vi "ConcidenceTesting.vi"() -> ()   [LabVIEW 2009]
panel:
  in  "new dim":cluster{"x":u32, "y":u32}={"x"=1, "y"=1}
  in  "re-calculate":bool
  in  "Palette Number (gray)":T1(ring)
  in  "coincidence settings":T2={"length [µs]"=10.0, "delayed channel"=0, "center peak (µs)"=0.5, "lateral peaks"=6} {"center peak (µs)" format="%.2f"; "length [µs]" format="%.2f"}
  in  "ratio":bool
  in  "threshold":u32
  in  "calculate":bool
  in  "including +/- Pixel":i32
  in  "stop":bool
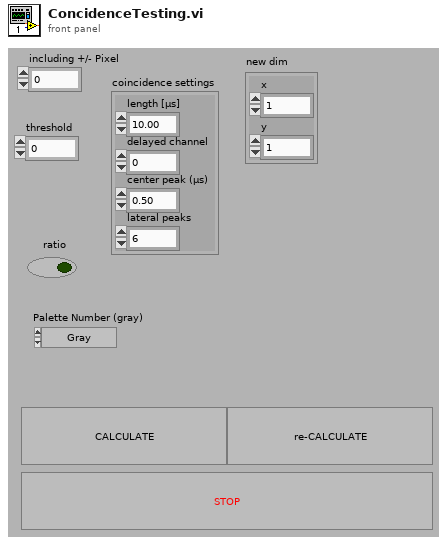
[diagram p1: front panel]
types:
  T1 = enum32{"Gray", "Binary", "Gradient", "Rainbow", "Temperature"}
  T2 = cluster{"length [µs]":dbl, "delayed channel":u8, "center peak (µs)":dbl, "lateral peaks":u32}
  T3 = enum16{"Ini", "Get", "Set", "Draw", "Colorpal", "Dump", "Zoom"}
  T4 = cluster{"router":u8[], "macro times":dbl[], "micro times":u16[], "invalid":dbl[], "gap":dbl[]}
  T5 = cluster{"origin (ns)":dbl, "offset (ns)":dbl, "histogram":u32[]}
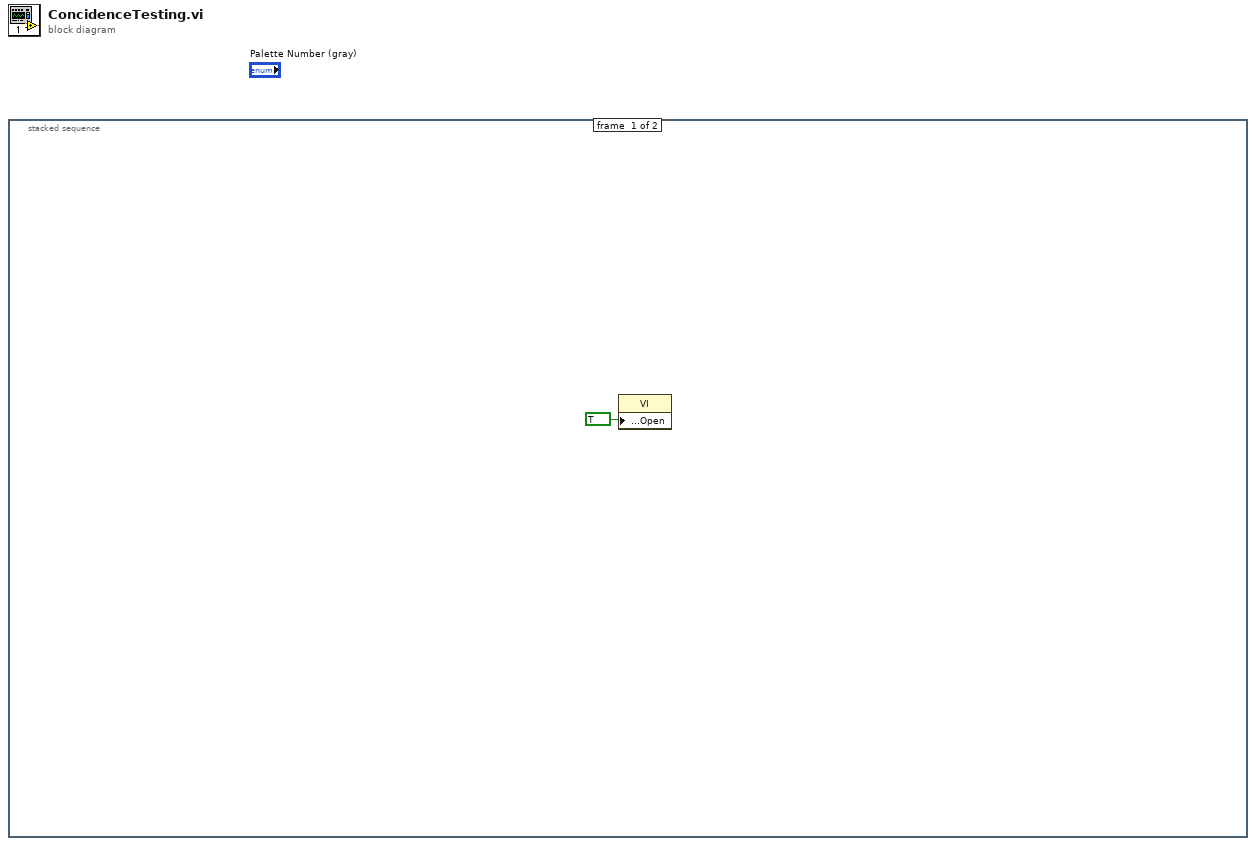
[diagram p0: block diagram]
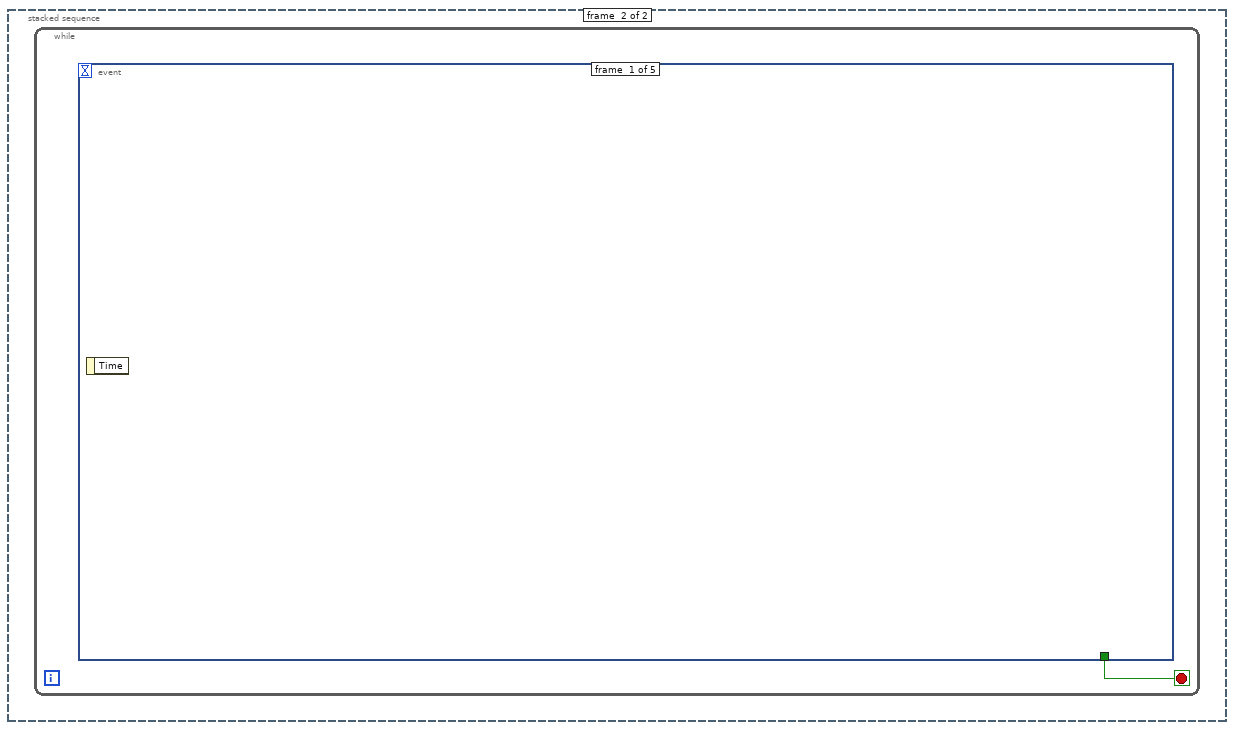
[diagram p2: hidden frame]
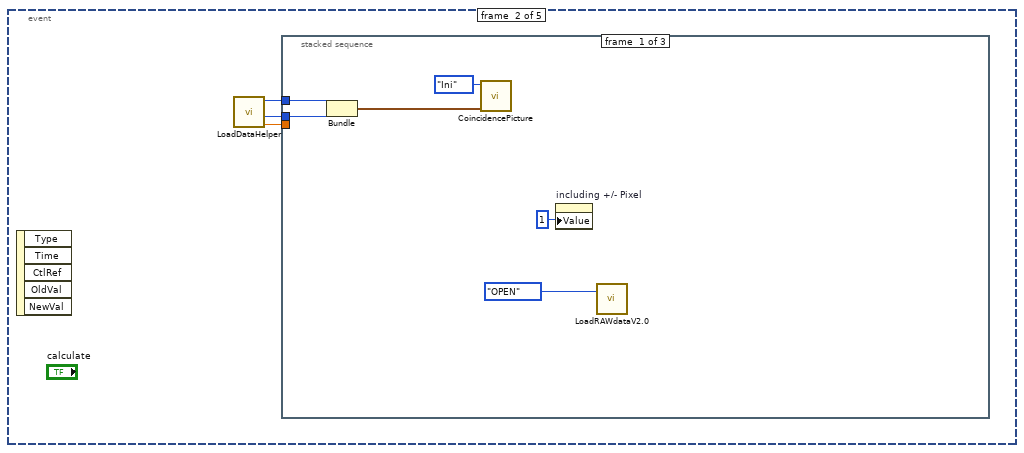
[diagram p3: hidden frame]
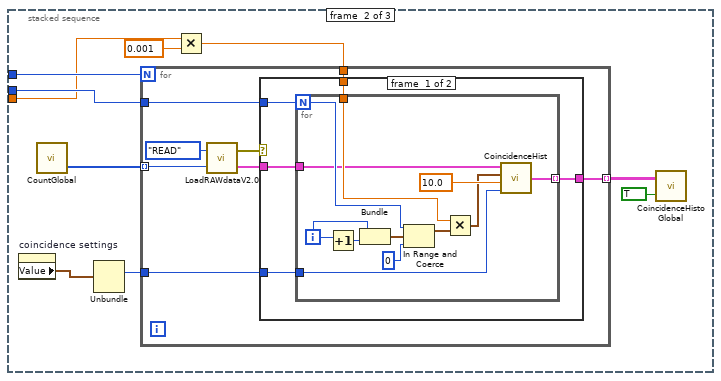
[diagram p4: hidden frame]
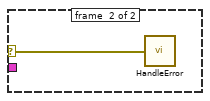
[diagram p5: hidden frame]
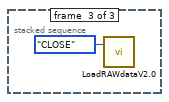
[diagram p6: hidden frame]
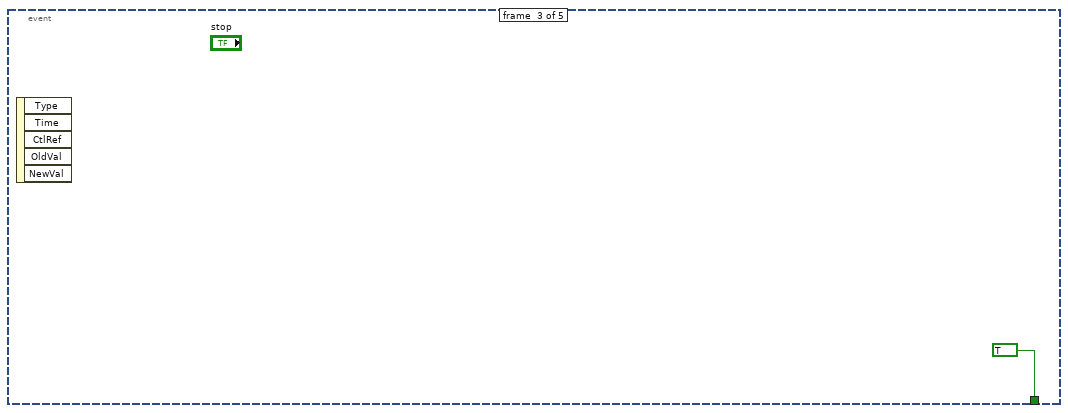
[diagram p7: hidden frame]
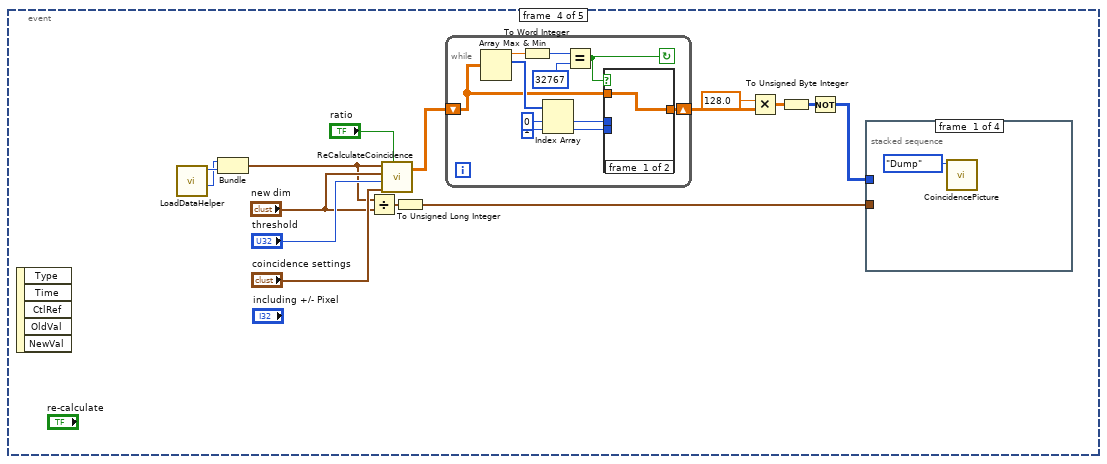
[diagram p8: hidden frame]
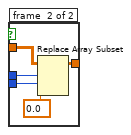
[diagram p9: hidden frame]
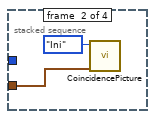
[diagram p10: hidden frame]
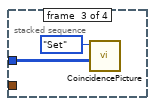
[diagram p11: hidden frame]
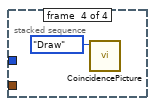
[diagram p12: hidden frame]
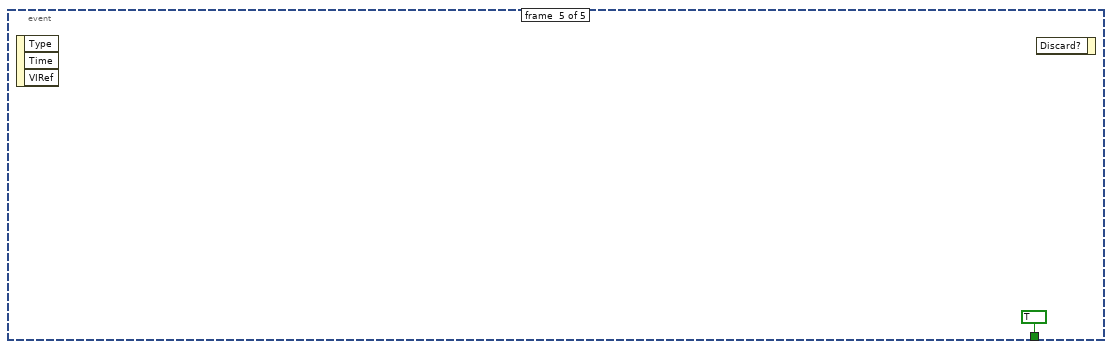
[diagram p13: hidden frame]
diagram:
  n1 = stacked-sequence {
    frame #0 {
      n2 = property class="VI"("Front Panel Window:Open"=TRUE) -> ()  [unwired: 2 in, 2 out]
    }
    frame #1 {
      n3 = while {
        stop <- w2 stop-if-true
        n4 = event shown="[3] \"re-calculate\", \"including +/- Pixel\", \"ratio\", \"threshold\", \"coincidence settings.center peak (µs)\", \"coincidence settings.lateral peaks\": Value Change" {
          selector: _ -> [_ _ _ _ _]
          dyn-events: _ -> [_ _ _ _ _]
          timeout: _ -> [_ _ _ _ _]
          tunnel: [_ _ TRUE _ TRUE] -> w2
          event #0 {
            n5 = event-data() -> ()  [unwired: 1 in, 1 out]
          }
          event #1 {
            n6 = event-data() -> ()  [unwired: 1 in, 5 out]
            n7 = call "LoadDataHelper.vi"() -> ("Time Resolution [ms/pixel]"=w3:dbl, "pixel per line"=w4:u32, "lines"=w5:u32)  [unwired: 7 in, 2 out]
            n8 = stacked-sequence {
              tunnel: w5 -> [w9 w18 _]
              tunnel: w4 -> [w8 w17 _]
              tunnel: w3 -> [_ w16 _]
              frame #0 {
                n9 = Bundle("lines"=w9, "pixel per line"=w8) -> (w7:cluster{"lines":u32, "pixel per line":u32})  [unwired: 1 in]
                n10 = call "CoincidencePicture.vi"("new IMAGElsize"=w7, "Enum"=T3."Ini") -> ()  [unwired: 5 in, 3 out]
                n11 = property on="including +/- Pixel" class="Digital (strict)"("Value"=1 ("including +/- Pixel")) -> ()  [unwired: 2 in, 2 out]
                n12 = call "LoadRAWdataV2.0.vi"("action"=enum16{"OPEN", "READ", "CLOSE"}."OPEN" ("Enum")) -> ()  [unwired: 1 in, 2 out]
              }
              frame #1 {
                n13 = property on="coincidence settings" class="Clust (strict)"() -> ("Value"=w13:T2)  [unwired: 2 in, 2 out]
                n14 = call "CountGlobal.vi"() -> ("count out"=w20:i32[])  [unwired: 3 in]
                n15 = Unbundle(w13) -> ("delayed channel"=w12:u8)  [unwired: 3 out]
                n16 = Multiply(x=w16, y=0.001) -> (x*y=w19:dbl)
                n17 = for {
                  N: w18 -> [_]
                  tunnel: w17 -> [w29]
                  tunnel: w20 -> [w28] mode=indexing
                  tunnel: w12 -> [w24]
                  tunnel: w19 -> [w23]
                  tunnel: [w22] -> w15 mode=indexing
                  n18 = call "LoadRAWdataV2.0.vi"("pos offset (0)"=w28, "action"=enum16{"OPEN", "READ", "CLOSE"}."READ" ("Enum")) -> ("RAW data"=w26:T4, "error out"=w25:errorcluster)
                  n19 = case shown="No Error" w25 {
                    selector: w25 -> [_ w47]
                    tunnel: w29 -> [w34 _]
                    tunnel: w26 -> [w31 _]
                    tunnel: w24 -> [w33 _]
                    tunnel: w23 -> [w32 _]
                    tunnel: [w30 _] -> w22
                    frame #0 {
                      n20 = for {
                        N: w34 -> [w41]
                        tunnel: w31 -> [w39]
                        tunnel: w33 -> [w46]
                        tunnel: w32 -> [w42]
                        tunnel: [w38] -> w30 mode=indexing
                        i -> [w35]
                        n21 = Increment(x=w35) -> (x+1=w36:i32)
                        n22 = Bundle(w35, w36) -> (w45:cluster{i32, i32})  [unwired: 1 in]
                        n23 = In Range and Coerce(upper limit=w41, x=w45, lower limit=0) -> (coerced(x)=w43:cluster{i32, i32})  [unwired: 1 out]
                        n24 = Multiply(x=w42, y=w43) -> (x*y=w37:cluster{dbl, dbl})
                        n25 = call "CoincidenceHist.vi"("delayed channel"=w46, "length (µs)"=10.0, "range"=w37, "input rawdata"=w39) -> ("coincidence histogram"=w38:T5)
                      }
                    }
                    frame #1 {
                      n26 = call "HandleError.vi"("error in (no error)"=w47) -> ()
                    }
                  }
                }
                n27 = call "CoincidenceHistoGlobal.vi"("set/change"=TRUE, "Array 2"=w15) -> ()  [unwired: 1 out]
              }
              frame #2 {
                n28 = call "LoadRAWdataV2.0.vi"("action"=enum16{"OPEN", "READ", "CLOSE"}."CLOSE" ("Enum")) -> ()  [unwired: 1 in, 2 out]
              }
            }
          }
          event #2 {
            n29 = event-data() -> ()  [unwired: 1 in, 5 out]
          }
          event #3 {
            n30 = event-data() -> ()  [unwired: 1 in, 5 out]
            n31 = call "LoadDataHelper.vi"() -> ("pixel per line"=w63:u32, "lines"=w64:u32)  [unwired: 7 in, 3 out]
            n32 = Bundle("pixel per line"=w63, "lines"=w64) -> (w52:cluster{"pixel per line":u32, "lines":u32})  [unwired: 1 in]
            n33 = Divide(x=w52, y="new dim") -> (x/y=w51:cluster{dbl, dbl})
            n34 = call "ReCalculateCoincidence.vi"("orig dim"=w52, "new dim"="new dim", "threshold"="threshold", "coincidence settings"="coincidence settings", "ratio"="ratio") -> ("output"=w55:dbl[][])  [unwired: 1 in]
            n35 = To Unsigned Long Integer(number=w51) -> (unsigned 32bit integer=w50:cluster{u32, u32})
            n36 = while {
              shift-right: [w65] -> w57
              shift-left: w55 -> [w66]
              stop <- w72 continue-if-true
              n37 = Array Max & Min(array=w66) -> (max value=w75:dbl, max index (indices)=w71:i32[])  [unwired: 2 out]
              n38 = To Word Integer(number=w75) -> (16bit integer=w73:i16)
              n39 = Index Array(array=w71, index #1=0 ("index"), index #2=1 ("index")) -> (element #1=w68:i32, element #2=w67:i32)
              n40 = Equal?(x=w73, y=i16 32767) -> (x = y?=w72:bool)
              n41 = case shown="True" w72 {
                tunnel: w66 -> [w76 w81]
                tunnel: w68 -> [_ w80]
                tunnel: w67 -> [_ w79]
                tunnel: [w76 w77] -> w65
                frame #0 {
                }
                frame #1 {
                  n42 = Replace Array Subset(array=w81, new element=0.0 ("new element/subarray"), index (row)=w80, index (col)=w79) -> (w77:dbl[][])
                }
              }
            }
            n43 = Multiply(x=128.0 ("y"), y=w57) -> (x*y=w59:dbl[][])
            n44 = To Unsigned Byte Integer(number=w59) -> (unsigned 8bit integer=w58:u8[][])
            n45 = Not(x=w58) -> (.not. x?=w54:u8[][])
            n46 = stacked-sequence {
              tunnel: w50 -> [_ w83 _ _]
              tunnel: w54 -> [_ _ w85 _]
              frame #0 {
                n47 = call "CoincidencePicture.vi"("Enum"=T3."Dump") -> ()  [unwired: 6 in, 3 out]
              }
              frame #1 {
                n48 = call "CoincidencePicture.vi"("new IMAGElsize"=w83, "Enum"=T3."Ini") -> ()  [unwired: 5 in, 3 out]
              }
              frame #2 {
                n49 = call "CoincidencePicture.vi"("Image Pixels (U8)"=w85, "Enum"=T3."Set") -> ()  [unwired: 5 in, 3 out]
              }
              frame #3 {
                n50 = call "CoincidencePicture.vi"("Enum"=T3."Draw") -> ()  [unwired: 6 in, 3 out]
              }
            }
          }
          event #4 {
            n51 = event-data() -> ()  [unwired: 1 in, 3 out]
            n52 = event-data() -> ()  [unwired: 2 in, 1 out]
          }
        }
      }
    }
  }
